vi "Read Waveform (Single).vi"(8 "error in (no error)":errorcluster, 9 "Maximum Time (5000 ms)":u32=5000, 10 "Channel (1: Channel 1)":u16(ring)=1 items=["Channel 1"=1, "Channel 2"=2, "Channel 3"=3, "Channel 4"=4], 11 "VISA resource name":refnum<visa-resource-name>) -> (0 "error out":errorcluster, 2 "Waveform Data":dbl[](graph), 3 "VISA resource name out":refnum<visa-resource-name>)   [LabVIEW 2015, in "ZhiYuan ZDS Series for TCP.lvlib"]
doc: "Initiates an acquisition on all channels that you enabled with the Configure Channel VI. The VI waits for the acquisition to complete and returns the waveform for the <B>Source Channel</B> you specified. If the oscilloscope did not complete the acquisition within the time period you specify with the <B>Timeout</B> control, the VI returns a timeout error. A common cause for a timeout error is the acquisition was not triggered. For example, the trigger level is out of range of the waveform.\n\nCall the Fetch Waveform VI to obtain the waveforms for each of the remaining enabled <B>Source Channels</B> without initiating another acquisition.\n\n<B>Note:</B> If your instrument does not support auto compensation for probe attenuation, you may need to adjust the scaling of the Waveform Data accordingly. This is handled automatically in the <B>Configure Channel</B> VI or can be done manually by multiplying the <B>Waveform Data</B> by the probe attenuation."
uses:
  ZhiYuan ZDS Series for TCP.lvlib
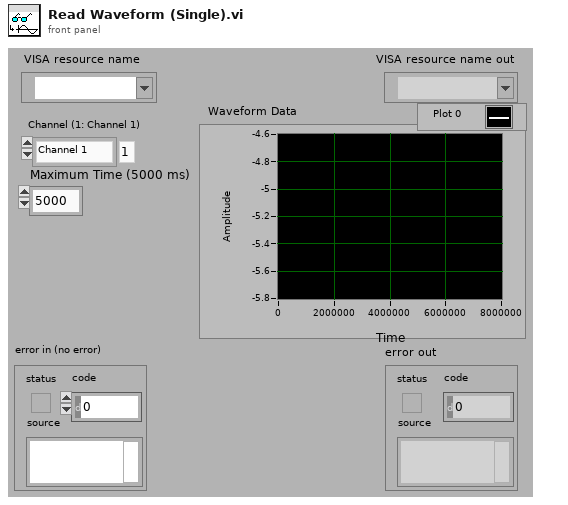
[diagram p1: front panel]
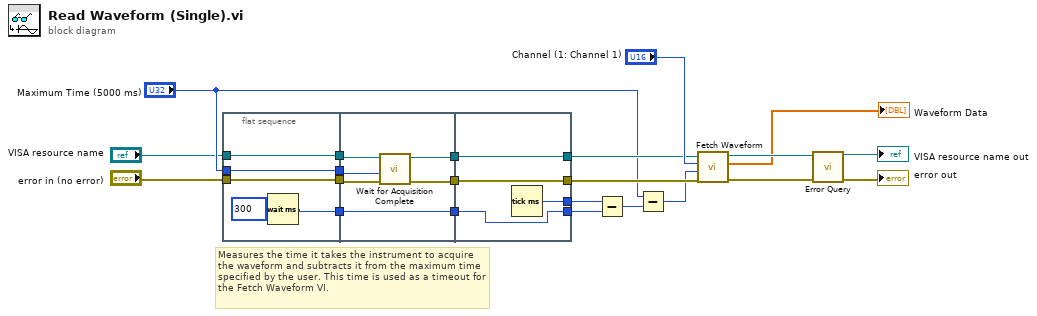
[diagram p0: block diagram]
diagram:
  # "Measures the time it takes the instrument to acquire the waveform and subtracts it from the maximum time specified by the user. This time is used as a timeout for the Fetch Waveform VI."
  n1 = flat-sequence {
    tunnel: "VISA resource name" -> [w27]
    tunnel: [w27] -> w9
    tunnel: "error in (no error)" -> [w26]
    tunnel: [w26] -> w8
    tunnel: "Maximum Time (5000 ms)" -> [w25]
    tunnel: [w25] -> w7
    tunnel: [w23] -> w6
    tunnel: w9 -> [w33]
    tunnel: [w32] -> w5
    tunnel: w8 -> [w31]
    tunnel: [w30] -> w4
    tunnel: w7 -> [w29]
    tunnel: w6 -> [w28]
    tunnel: [w28] -> w3
    tunnel: [w36] -> w16
    tunnel: w5 -> [w36]
    tunnel: [w35] -> w15
    tunnel: w4 -> [w35]
    tunnel: [w34] -> w11
    tunnel: w3 -> [w34]
    tunnel: [w37] -> w10
    frame #0 {
      n2 = Wait (ms)(milliseconds to wait=300) -> (millisecond timer value=w23:u32)
    }
    frame #1 {
      n3 = call "Wait for Acquisition Complete.vi"("error in (no error)"=w31, "Maximum Time (10000 ms)"=w29, "VISA resource name"=w33) -> ("error out"=w30:errorcluster, "VISA resource name out"=w32:refnum<visa-resource-name>)  [unwired: 7 in]
    }
    frame #2 {
      n4 = Tick Count (ms)() -> (millisecond timer value=w37:u32)
    }
  }
  n5 = Subtract(x=w10, y=w11) -> (x-y=w14:u32)
  n6 = Subtract(x="Maximum Time (5000 ms)", y=w14) -> (x-y=w12:u32)
  n7 = call "Fetch Waveform.vi"("error in (no error)"=w15, "Timeout (5000 ms)"=w12, "Channel (1: Channel 1)"="Channel (1: Channel 1)", "VISA resource name"=w16) -> ("error out"=w18:errorcluster, "Waveform Data"=→"Waveform Data":dbl[], "VISA resource name out"=w19:refnum<visa-resource-name>)  [unwired: 5 in]
  n8 = call "Error Query.vi"("error in (no error)"=w18, "VISA resource name"=w19) -> ("error out"=→"error out":errorcluster, "VISA resource name out"=→"VISA resource name out":refnum<visa-resource-name>)  [unwired: 6 in, 2 out]
